vi "Check_values_conversion.vi"(3 "Sampling Rate":dbl, 4 "Wait  Count":i32, 5 "Delay  Count":i32, 6 "Velocity  Count":i32) -> (0 "Wait time":dbl, 1 "Delay":dbl, 2 "Measured Velocity":dbl)   [LabVIEW 2015]
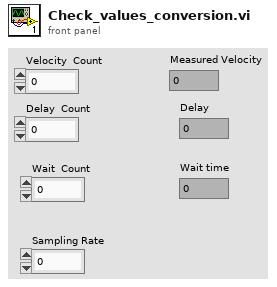
[diagram p1: front panel]
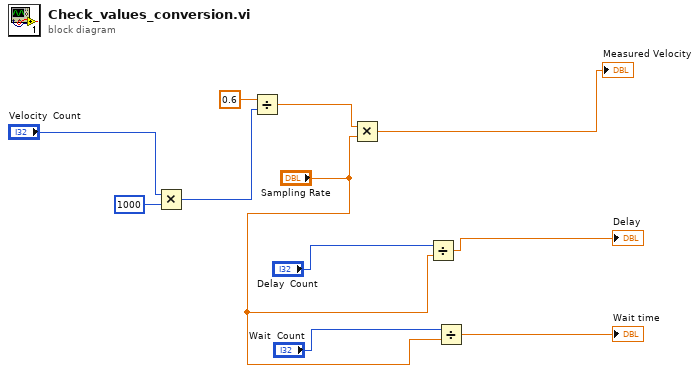
[diagram p0: block diagram]
diagram:
  n1 = Multiply(x="Velocity  Count", y=1000) -> (x*y=w9:i32)
  n2 = Divide(x=0.6, y=w9) -> (x/y=w10:dbl)
  n3 = Multiply(x=w10, y="Sampling Rate") -> (x*y=→"Measured Velocity":dbl)
  n4 = Divide(x="Delay  Count", y="Sampling Rate") -> (x/y=→"Delay":dbl)
  n5 = Divide(x="Wait  Count", y="Sampling Rate") -> (x/y=→"Wait time":dbl)
